vi "Test Generic Write.vi"() -> ()   [LabVIEW 2017]
uses:
  <vilib>/Rock Robotics/Network Tables/Field Data.ctl
  <vilib>/Rock Robotics/Network Tables/Field Type.ctl
  <vilib>/Rock Robotics/Network Tables/Sequence.ctl
panel:
  out "Field Value":T1
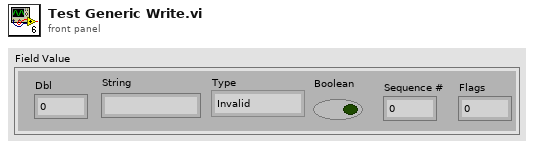
[diagram p1: front panel]
types:
  T1 = typedef "Field Data.ctl" = cluster{"Dbl":dbl, "String":string, "Type":T2, "Boolean":bool, "Sequence #":T3, "Flags":u8}
  T2 = typedef "Field Type.ctl" = enum8{"Invalid", "Bool", "Numeric", "String", "Raw", "Boolean Array", "Numeric Array", "String Array", "RPC"}
  T3 = typedef "Sequence.ctl" = u16
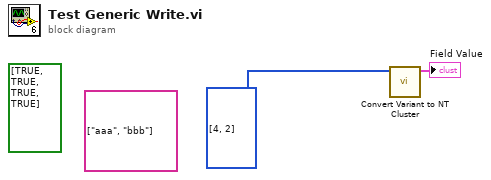
[diagram p0: block diagram]
diagram:
  (unwired) string[] ["aaa", "bbb"]
  (unwired) bool[] [TRUE, TRUE, TRUE, TRUE]
  n1 = call <vilib>:"Convert Variant to NT Cluster.vi"("NewVal"=u64[] [4, 2]) -> ("Field Value"=→"Field Value":T1)  [unwired: 10 in]
